vi "PIO_DIR.vi"(2 "error in (no error)":errorcluster, 3 "Output/Input":dbl min=0.0 max=1.0, 4 "Select Channel":dbl=1.0 min=1.0 max=6.0, 5 "VISA resource Input":refnum<visa-resource-name>) -> (0 "error out":errorcluster, 1 "VISA resource Quit":refnum<visa-resource-name>)   [LabVIEW 2011]
panel:
  out "unsigned byte array":u8[](array[numeric])
  out "return count":u32
  out "Read PIO_DIR command":u8[](array[numeric])
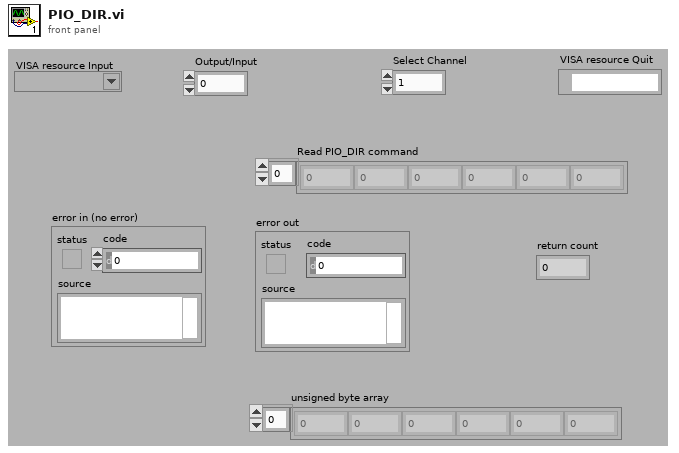
[diagram p1: front panel]
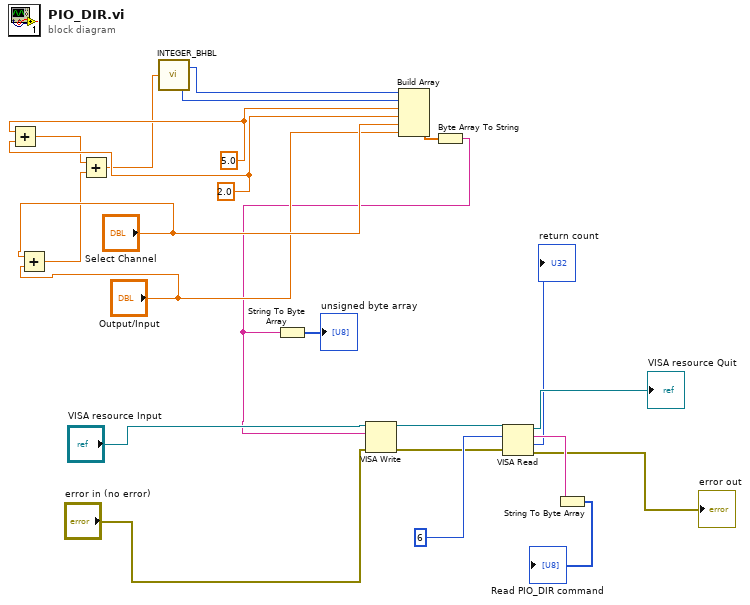
[diagram p0: block diagram]
diagram:
  w10 = 2.0 ("element")
  w11 = 5.0 ("element")
  n1 = Add(x=w11, y=w10) -> (x+y=w9:dbl)
  n2 = Add(x="Select Channel", y="Output/Input") -> (x+y=w6:dbl)
  n3 = Add(x=w9, y=w6) -> (x+y=w5:dbl)
  n4 = call "INTEGER_BHBL.vi"("int16"=w5) -> ("Lvalue"=w3:u8, "HValue"=w4:u8)
  n5 = Build Array(w4, w3, w11, w10, "Select Channel", "Output/Input") -> (w15:dbl[])
  n6 = Byte Array To String(unsigned byte array=w15) -> (string=w2:string)
  n7 = String To Byte Array(string=w2) -> (unsigned byte array=→"unsigned byte array":u8[])
  n8 = VISA Write(VISA resource name="VISA resource Input", write buffer=w2, error in (no error)="error in (no error)") -> (VISA resource name out=w16:refnum<visa-resource-name>, error out=w18:errorcluster)  [unwired: 1 out]
  n9 = VISA Read(VISA resource name=w16, byte count=u32 6, error in (no error)=w18) -> (VISA resource name out=→"VISA resource Quit":refnum<visa-resource-name>, read buffer=w21:string, return count=→"return count":u32, error out=→"error out":errorcluster)
  n10 = String To Byte Array(string=w21) -> (unsigned byte array=→"Read PIO_DIR command":u8[])
